vi "hModeRegRange2013.vi"(4 "error in":errorcluster, 5 "RangeArray":u8[](array[numeric]), 6 "Mode":u16 format="%x", 7 "FPGA VI Reference In":refnum<k20>) -> (0 "error out":errorcluster, 2 "Timeout":bool, 3 "FPGA VI Reference Out":refnum<k20>)   [LabVIEW 2014]
doc: "Schreibt eine gemeinsame Konfiguration in alle Moderegister."
panel:
  out "dimens":u8=24
  out "boll arr":bool[](array[boolean])
  out "long bool arr":bool[](array[boolean])
  out "write array to host write":u32
  out "hex * range":u8
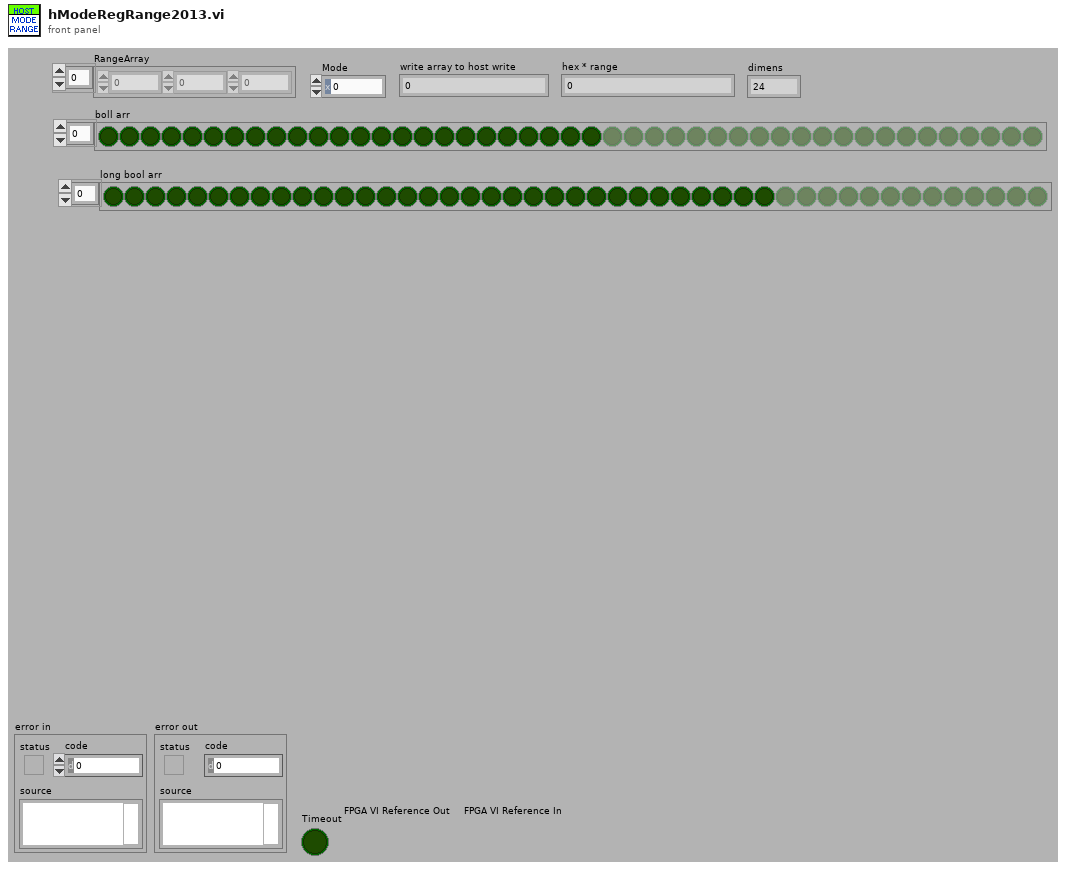
[diagram p1: front panel]
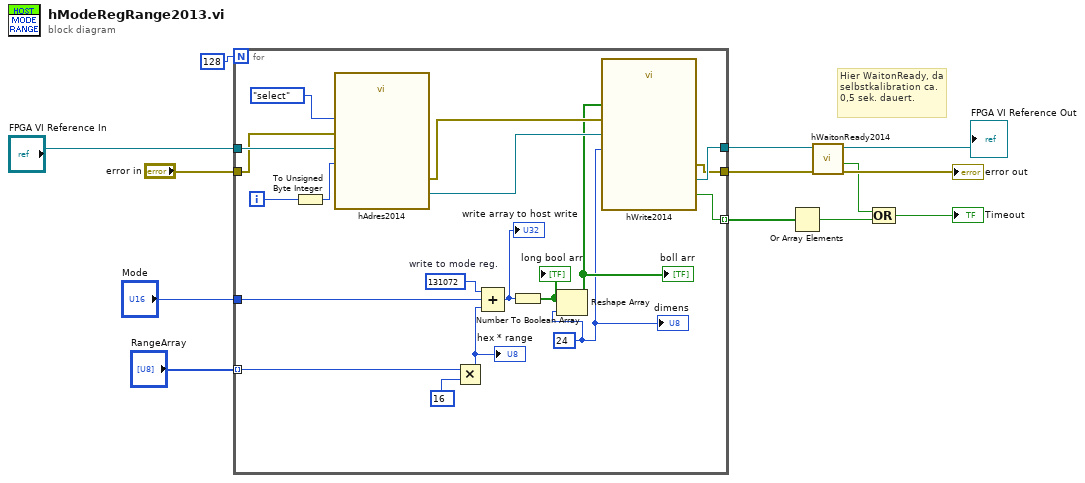
[diagram p0: block diagram]
diagram:
  # "Hier WaitonReady, da selbstkalibration ca. 0,5 sek. dauert."
  n1 = for {
    N: 128 -> [_]
    tunnel: [w24] -> w10 mode=indexing
    tunnel: [w21] -> w9
    tunnel: [w20] -> w8
    tunnel: "FPGA VI Reference In" -> [w19]
    tunnel: "error in" -> [w18]
    tunnel: "RangeArray" -> [w17] mode=indexing
    tunnel: "Mode" -> [w16]
    i -> [w15]
    w31 = u32 131072  # write to mode reg.
    w22 = u8 24
    n2 = To Unsigned Byte Integer(number=w15) -> (unsigned 8bit integer=w14:u8)
    n3 = call "hAdres2014.vi"("error in"=w18, "Kanal#"=w14, "AdressMode"=enum16{"select", "oben", "unten", "keinen"}."select", "FPGA VI Reference In"=w19) -> ("error out"=w25:errorcluster, "FPGA VI Reference Out"=w26:refnum<k20>)  [unwired: 2 in]
    n4 = Multiply(x=w17, y=u8 16) -> (x*y=w29:u8)
    "hex * range" <- w29
    n5 = Compound Arithmetic op=unknown(w31, w16, w29) -> (w32:u32)
    "write array to host write" <- w32
    n6 = Number To Boolean Array(number=w32) -> (Boolean array=w30:bool[])
    "long bool arr" <- w30
    n7 = Reshape Array(w30, w22) -> (w23:bool[])
    "boll arr" <- w23
    n8 = call "hWrite2014.vi"("error in"=w25, "nbit"=w22, "Data"=w23, "FPGA VI Reference In"=w26) -> ("error out"=w20:errorcluster, "Timed Out"=w24:bool, "FPGA VI Reference Out"=w21:refnum<k20>)  [unwired: 1 in]
    "dimens" <- w22
  }
  n9 = Or Array Elements(Boolean array=w10) -> (logical OR=w4:bool)
  n10 = call "hWaitonReady2014.vi"("error in"=w8, "FPGA VI Reference In"=w9) -> ("error out"=→"error out":errorcluster, "Timeout"=w12:bool, "FPGA VI Reference Out"=→"FPGA VI Reference Out":refnum<k20>)  [unwired: 3 in]
  n11 = Compound Arithmetic op=OR(w12, w4) -> (→"Timeout":bool)
